vi "APC_9056_ErrorMask.vi"(7 "SYSTEM STATE":i8=3) -> (4 "raster1mask":bool[](array[boolean])=[TRUE, TRUE, TRUE, TRUE, TRUE, TRUE, TRUE, TRUE, TRUE, TRUE, TRUE, TRUE, TRUE, TRUE, TRUE, TRUE], 6 "raster2mask":bool[](array[boolean])=[TRUE, TRUE, TRUE, TRUE, TRUE, TRUE, TRUE, TRUE, TRUE, TRUE, TRUE, TRUE, TRUE, TRUE, TRUE, TRUE], 8 "raster3mask":bool[](array[boolean])=[TRUE, TRUE, TRUE, TRUE, TRUE, TRUE, TRUE, TRUE, TRUE, TRUE, TRUE, TRUE, TRUE, TRUE, TRUE, TRUE], 10 "raster4mask":bool[](array[boolean])=[TRUE, TRUE, TRUE, TRUE, TRUE, TRUE, TRUE, TRUE, TRUE, TRUE, TRUE, TRUE, TRUE, TRUE, TRUE, TRUE], 13 "CylinderMask":bool[](array[boolean]), 15 "raster5mask":bool[](array[boolean])=[TRUE, TRUE, TRUE, TRUE, TRUE, TRUE, TRUE, TRUE, TRUE, TRUE, TRUE, TRUE, TRUE, TRUE, TRUE, TRUE])   [LabVIEW 2020]
panel:
  in  "Firing (3)":bool[](array[boolean])=[TRUE, FALSE, FALSE, TRUE, FALSE]
  in  "Idling (2)":bool[](array[boolean])=[TRUE, FALSE, FALSE, TRUE, FALSE]
  in  "Motoring (1)":bool[](array[boolean])=[FALSE, FALSE, FALSE, FALSE, FALSE]
  in  "Standby (0)":bool[](array[boolean])=[FALSE, FALSE, FALSE, FALSE, FALSE]
  in  "Safe mode (-1)":bool[](array[boolean])=[FALSE, FALSE, FALSE, FALSE, FALSE]
  in  "ACTIVE ERRORS FOR LOW SPEED":bool[][](array[boolean])=[[TRUE, TRUE, TRUE, TRUE, TRUE], [TRUE, TRUE, TRUE, TRUE, TRUE], [TRUE, TRUE, TRUE, TRUE, TRUE], [TRUE, TRUE, TRUE, TRUE, TRUE], [TRUE, TRUE, TRUE, TRUE, TRUE], [TRUE, TRUE, TRUE, TRUE, TRUE], [TRUE, TRUE, TRUE, TRUE, TRUE], [TRUE, TRUE, TRUE, TRUE, TRUE], [TRUE, TRUE, TRUE, TRUE, TRUE], [TRUE, TRUE, TRUE, TRUE, TRUE], [TRUE, TRUE, TRUE, TRUE, TRUE], [TRUE, TRUE, TRUE, TRUE, TRUE], [TRUE, TRUE, TRUE, TRUE, TRUE], [TRUE, TRUE, TRUE, TRUE, TRUE], [TRUE, TRUE, TRUE, TRUE, TRUE], [TRUE, TRUE, TRUE, TRUE, TRUE]]
  in  "MinEngineSpeedforMask":dbl=1000.0
  in  "EngineSpeed":dbl
  in  "Firing (3)":bool[][](array[boolean])=[[TRUE, TRUE, TRUE, TRUE, TRUE], [TRUE, TRUE, TRUE, TRUE, TRUE], [TRUE, TRUE, TRUE, TRUE, TRUE], [TRUE, TRUE, TRUE, TRUE, TRUE], [TRUE, TRUE, TRUE, TRUE, TRUE], [TRUE, TRUE, TRUE, TRUE, TRUE], [TRUE, TRUE, TRUE, TRUE, TRUE], [TRUE, TRUE, TRUE, TRUE, TRUE], [TRUE, TRUE, TRUE, TRUE, TRUE], [TRUE, TRUE, TRUE, TRUE, TRUE], [TRUE, TRUE, TRUE, TRUE, TRUE], [TRUE, TRUE, TRUE, TRUE, TRUE], [TRUE, TRUE, TRUE, TRUE, TRUE], [TRUE, TRUE, TRUE, TRUE, TRUE], [TRUE, TRUE, TRUE, TRUE, TRUE], [TRUE, TRUE, TRUE, TRUE, TRUE]]
  in  "Idling (2)":bool[][](array[boolean])=[[TRUE, TRUE, TRUE, TRUE, TRUE], [TRUE, TRUE, TRUE, TRUE, TRUE], [TRUE, TRUE, TRUE, TRUE, TRUE], [TRUE, TRUE, TRUE, TRUE, TRUE], [TRUE, TRUE, TRUE, TRUE, TRUE], [TRUE, TRUE, TRUE, TRUE, TRUE], [TRUE, TRUE, TRUE, TRUE, TRUE], [TRUE, TRUE, TRUE, TRUE, TRUE], [TRUE, TRUE, TRUE, TRUE, TRUE], [TRUE, TRUE, TRUE, TRUE, TRUE], [TRUE, TRUE, TRUE, TRUE, TRUE], [TRUE, TRUE, TRUE, TRUE, TRUE], [TRUE, TRUE, TRUE, TRUE, TRUE], [TRUE, TRUE, TRUE, TRUE, TRUE], [TRUE, TRUE, TRUE, TRUE, TRUE], [TRUE, TRUE, TRUE, TRUE, TRUE]]
  in  "Motoring (1)":bool[][](array[boolean])=[[TRUE, TRUE, TRUE, TRUE, TRUE], [TRUE, TRUE, TRUE, TRUE, TRUE], [TRUE, TRUE, TRUE, TRUE, TRUE], [TRUE, TRUE, TRUE, TRUE, TRUE], [TRUE, TRUE, TRUE, TRUE, TRUE], [TRUE, TRUE, TRUE, TRUE, TRUE], [TRUE, TRUE, TRUE, TRUE, TRUE], [TRUE, TRUE, TRUE, TRUE, TRUE], [TRUE, TRUE, TRUE, TRUE, TRUE], [TRUE, TRUE, TRUE, TRUE, TRUE], [TRUE, TRUE, TRUE, TRUE, TRUE], [TRUE, TRUE, TRUE, TRUE, TRUE], [TRUE, TRUE, TRUE, TRUE, TRUE], [TRUE, TRUE, TRUE, TRUE, TRUE], [TRUE, TRUE, TRUE, TRUE, TRUE], [TRUE, TRUE, TRUE, TRUE, TRUE]]
  in  "Standby (0)":bool[][](array[boolean])=[[FALSE, FALSE, FALSE, FALSE, FALSE], [FALSE, FALSE, FALSE, FALSE, FALSE], [FALSE, FALSE, FALSE, FALSE, FALSE], [FALSE, FALSE, FALSE, FALSE, FALSE], [FALSE, FALSE, FALSE, FALSE, FALSE], [FALSE, FALSE, FALSE, FALSE, FALSE], [FALSE, FALSE, FALSE, FALSE, FALSE], [FALSE, FALSE, FALSE, FALSE, FALSE], [FALSE, FALSE, FALSE, FALSE, FALSE], [FALSE, FALSE, FALSE, FALSE, FALSE], [FALSE, FALSE, FALSE, FALSE, FALSE], [FALSE, FALSE, FALSE, FALSE, FALSE], [FALSE, FALSE, FALSE, FALSE, FALSE], [FALSE, FALSE, FALSE, FALSE, FALSE], [FALSE, FALSE, FALSE, FALSE, FALSE], [FALSE, FALSE, FALSE, FALSE, FALSE]]
  in  "Safe mode (-1)":bool[][](array[boolean])=[[FALSE, FALSE, FALSE, FALSE, FALSE], [FALSE, FALSE, FALSE, FALSE, FALSE], [FALSE, FALSE, FALSE, FALSE, FALSE], [FALSE, FALSE, FALSE, FALSE, FALSE], [FALSE, FALSE, FALSE, FALSE, FALSE], [FALSE, FALSE, FALSE, FALSE, FALSE], [FALSE, FALSE, FALSE, FALSE, FALSE], [FALSE, FALSE, FALSE, FALSE, FALSE], [FALSE, FALSE, FALSE, FALSE, FALSE], [FALSE, FALSE, FALSE, FALSE, FALSE], [FALSE, FALSE, FALSE, FALSE, FALSE], [FALSE, FALSE, FALSE, FALSE, FALSE], [FALSE, FALSE, FALSE, FALSE, FALSE], [FALSE, FALSE, FALSE, FALSE, FALSE], [FALSE, FALSE, FALSE, FALSE, FALSE], [FALSE, FALSE, FALSE, FALSE, FALSE]]
  # "MaxPressure"
  # "Misfire"
  # "Cyclic variability"
  # "Knock"
  # "Late combustion"
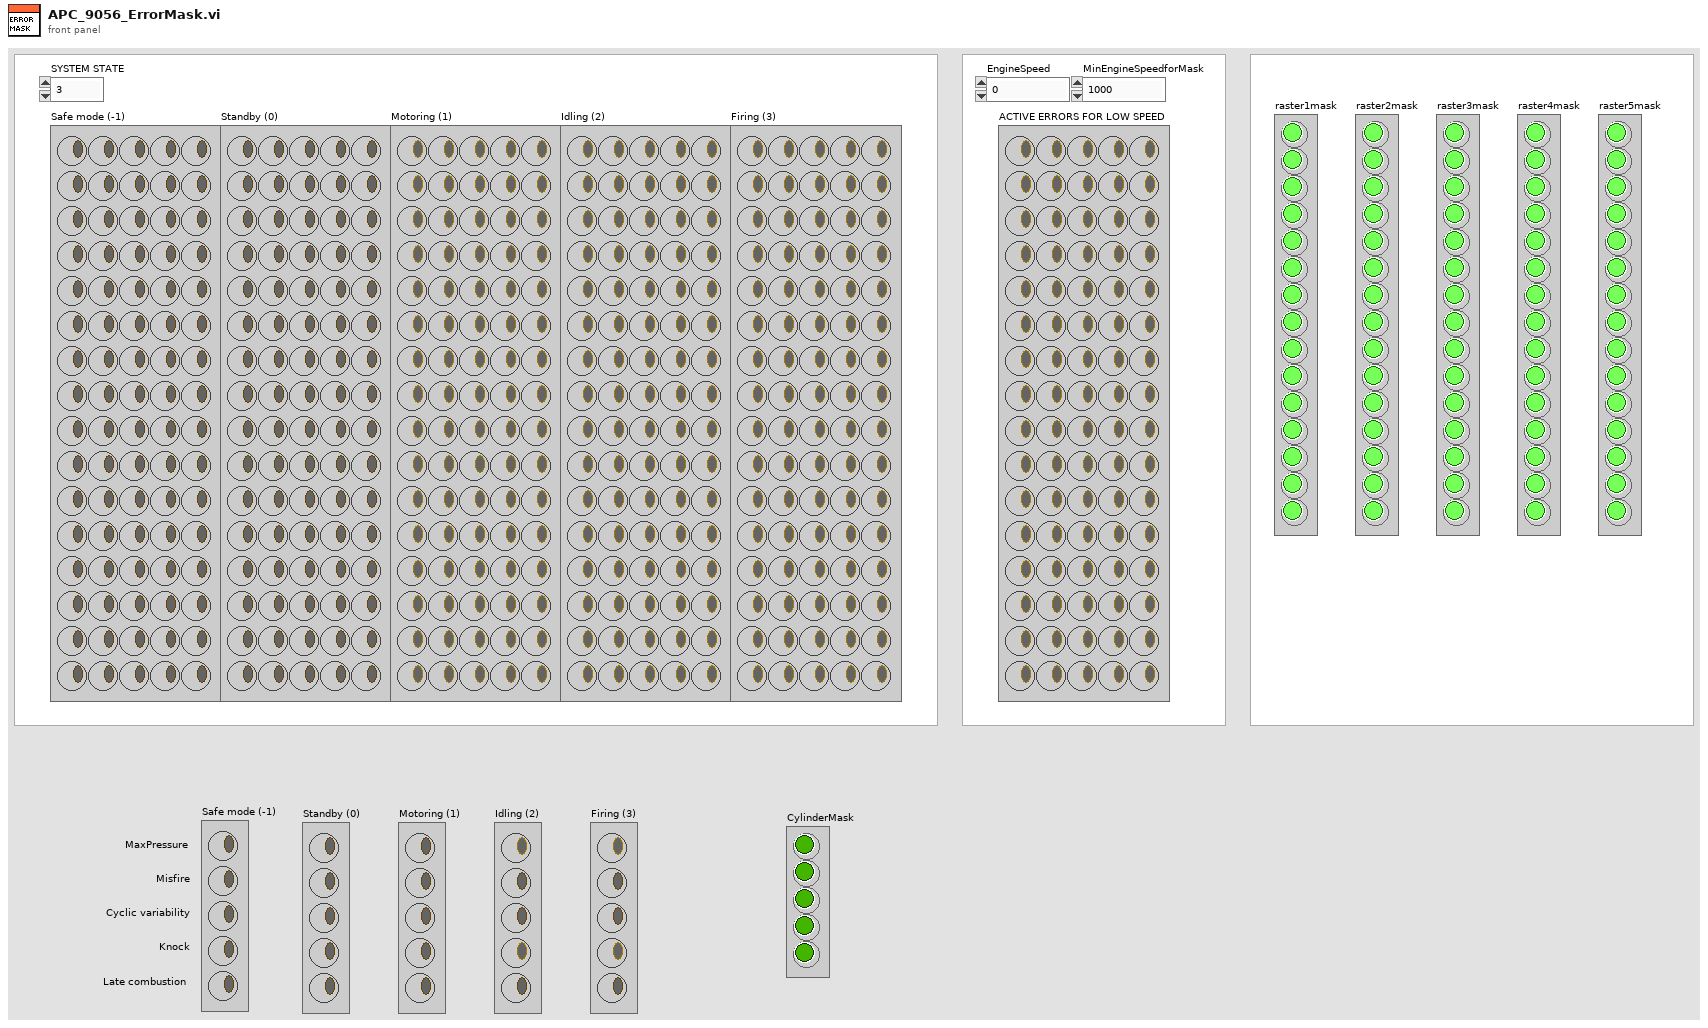
[diagram p1: front panel]
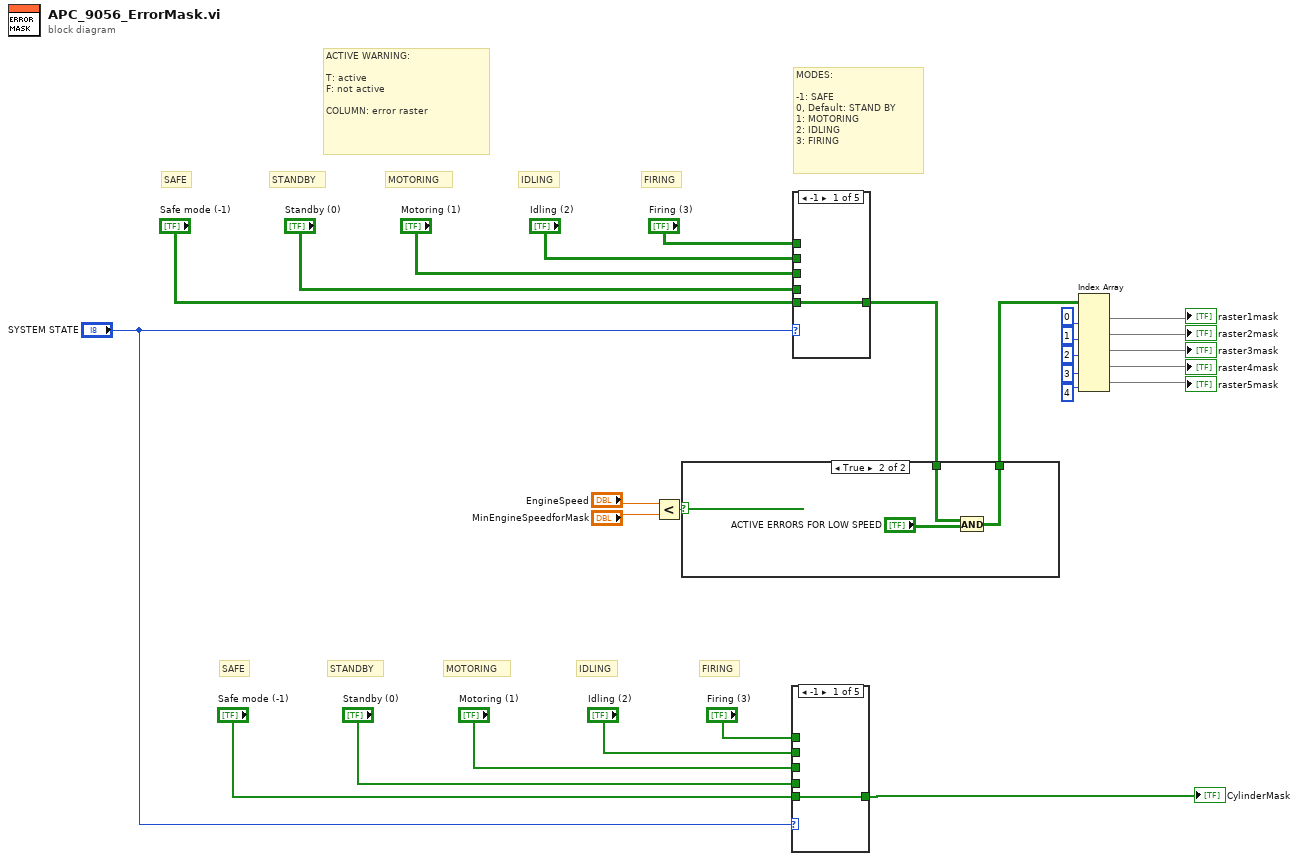
[diagram p0: block diagram]
diagram:
  # "FIRING"
  # "IDLING"
  # "MOTORING"
  # "STANDBY"
  # "SAFE"
  # "FIRING"
  # "IDLING"
  # "MOTORING"
  # "STANDBY"
  # "SAFE"
  # "ACTIVE WARNING:\n\nT: active\nF: not active \n\nCOLUMN: error raster"
  # "MODES:\n\n-1: SAFE\n0, Default: STAND BY\n1: MOTORING\n2: IDLING\n3: FIRING"
  n1 = Less?(x="EngineSpeed", y="MinEngineSpeedforMask") -> (x < y?=w10:bool)
  n2 = case shown="-1" "SYSTEM STATE" {
    tunnel: "Safe mode (-1)" -> [w28 _ _ _ _]
    tunnel: "Standby (0)" -> [_ w29 _ _ _]
    tunnel: "Motoring (1)" -> [_ _ w30 _ _]
    tunnel: "Idling (2)" -> [_ _ _ w31 _]
    tunnel: "Firing (3)" -> [_ _ _ _ w32]
    tunnel: [w28 w29 w30 w31 w32] -> w1
    frame -1 {
    }
    frame 0, Default {
    }
    frame 1 {
    }
    frame 2 {
    }
    frame 3 {
    }
  }
  "CylinderMask" <- w1
  n3 = case shown="-1" "SYSTEM STATE" {
    tunnel: "Safe mode (-1)" -> [w33 _ _ _ _]
    tunnel: "Standby (0)" -> [_ w34 _ _ _]
    tunnel: "Motoring (1)" -> [_ _ w35 _ _]
    tunnel: "Idling (2)" -> [_ _ _ w36 _]
    tunnel: "Firing (3)" -> [_ _ _ _ w37]
    tunnel: [w33 w34 w35 w36 w37] -> w9
    frame -1 {
    }
    frame 0, Default {
    }
    frame 1 {
    }
    frame 2 {
    }
    frame 3 {
    }
  }
  n4 = case shown="True" w10 {
    tunnel: w9 -> [w38 w40]
    tunnel: [w38 w39] -> w8
    frame False {
    }
    frame True {
      n5 = And(x=w40, y="ACTIVE ERRORS FOR LOW SPEED") -> (x .and. y?=w39:bool[][])
    }
  }
  n6 = Index Array(array=w8, index (col) #1=0 ("disabled index (col)"), index (col) #2=1 ("index (col)"), index (col) #3=2 ("index (col)"), index (col) #4=3 ("index (col)"), index (col) #5=4 ("index (col)")) -> (element #1=→"raster1mask":bool[], element #2=→"raster2mask":bool[], element #3=→"raster3mask":bool[], element #4=→"raster4mask":bool[], element #5=→"raster5mask":bool[])  [unwired: 5 in]
